vi "CRYSet All Editor Front Panel.vi"(11 "VI Ref":refnum<vi> caption="Vi Ref") -> ()   [LabVIEW 2013]
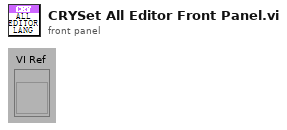
[diagram p1: front panel]
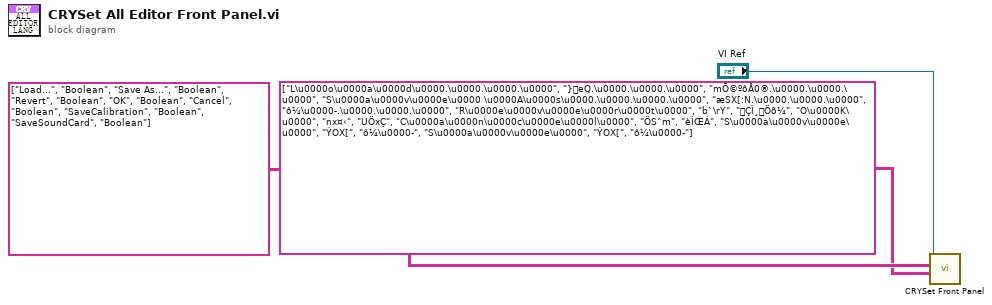
[diagram p0: block diagram]
diagram:
  n1 = call "CRYSet Front Panel.vi"("Caption(Boolean Text)"=string[][] [["L\u0000o\u0000a\u0000d\u0000.\u0000.\u0000.\u0000", "}eQ.\u0000.\u0000.\u0000", "mÕ©ºôÅ0®.\u0000.\u0000.\u0000"], ["S\u0000a\u0000v\u0000e\u0000 \u0000A\u0000s\u0000.\u0000.\u0000.\u0000", "æSX[:N.\u0000.\u0000.\u0000", "ô¼\u0000­.\u0000.\u0000.\u0000"], ["R\u0000e\u0000v\u0000e\u0000r\u0000t\u0000", "b`\rY", "ÇÌ¸Öõ¼"], ["O\u0000K\u0000", "nx¤‹", "UÖxÇ"], ["C\u0000a\u0000n\u0000c\u0000e\u0000l\u0000", "ÖSˆm", "èÍŒÁ"], ["S\u0000a\u0000v\u0000e\u0000", "ÝOX[", "ô¼\u0000­"], ["S\u0000a\u0000v\u0000e\u0000", "ÝOX[", "ô¼\u0000­"]], "Control ID and Type(Label Name, Type)"=string[][] [["Load...", "Boolean"], ["Save As...", "Boolean"], ["Revert", "Boolean"], ["OK", "Boolean"], ["Cancel", "Boolean"], ["SaveCalibration", "Boolean"], ["SaveSoundCard", "Boolean"]], "Vi Ref"="VI Ref") -> ()  [unwired: 9 in]
